vi "Serial Write.vi"(8 "error in (no error)":errorcluster, 10 "Input Command Frame":string, 11 "VISA resource name":refnum<visa-resource-name>) -> (0 "error out":errorcluster, 2 "Bytes Count":i32, 3 "VISA resource name out":refnum<visa-resource-name>)   [LabVIEW 2019, in "BK Precision 178XB Series.lvlib"]
doc: "This VI writes information through the serial port."
uses:
  BK Precision 178XB Series.lvlib
panel:
  in  "Communication Address":u8 max=254 format="%x"
  in  "Start":u8=170 format="%02x"
  in  "Command":u8 format="%02x"
  in  "B01":u8 format="%02x"
  in  "B02":u8 format="%02x"
  in  "B03":u8 format="%02x"
  in  "B04":u8 format="%02x"
  in  "B05":u8 format="%02x"
  in  "B06":u8 format="%02x"
  in  "B07":u8 format="%02x"
  in  "B08":u8 format="%02x"
  in  "B09":u8 format="%02x"
  in  "B10":u8 format="%02x"
  in  "B11":u8 format="%02x"
  in  "B12":u8 format="%02x"
  in  "B13":u8 format="%02x"
  in  "B14":u8 format="%02x"
  in  "B15":u8 format="%02x"
  in  "B16":u8 format="%02x"
  in  "B17":u8 format="%02x"
  in  "B18":u8 format="%02x"
  in  "B19":u8 format="%02x"
  in  "B20":u8 format="%02x"
  in  "B21":u8 format="%02x"
  in  "B22":u8 format="%02x"
  out "CS":u8 format="%02x"
  out "Output Command Frame":u8[](array[numeric])
  # "(c) 2009 B&K PRECISION CORPORATION.  ALL RIGHTS RESERVED."
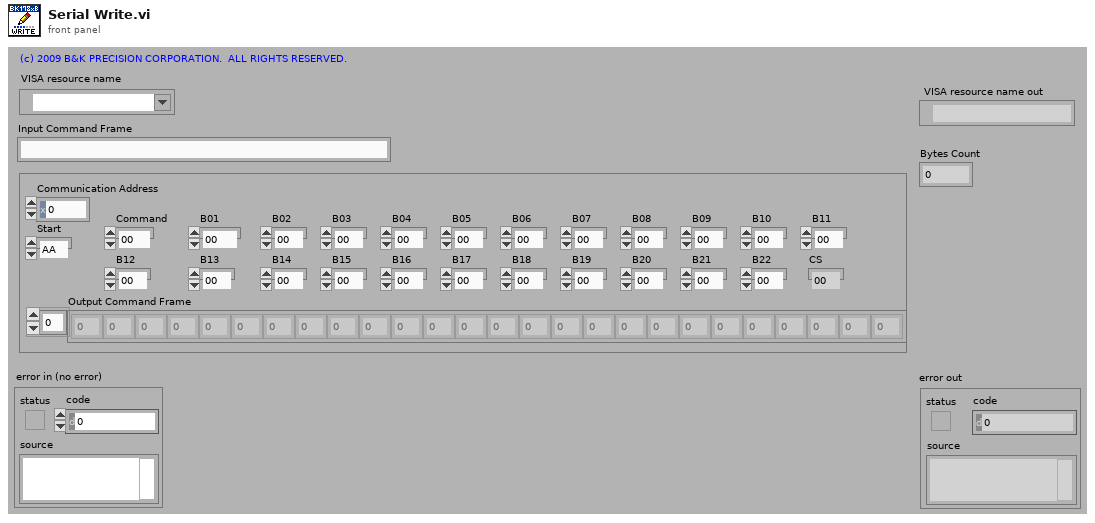
[diagram p1: front panel]
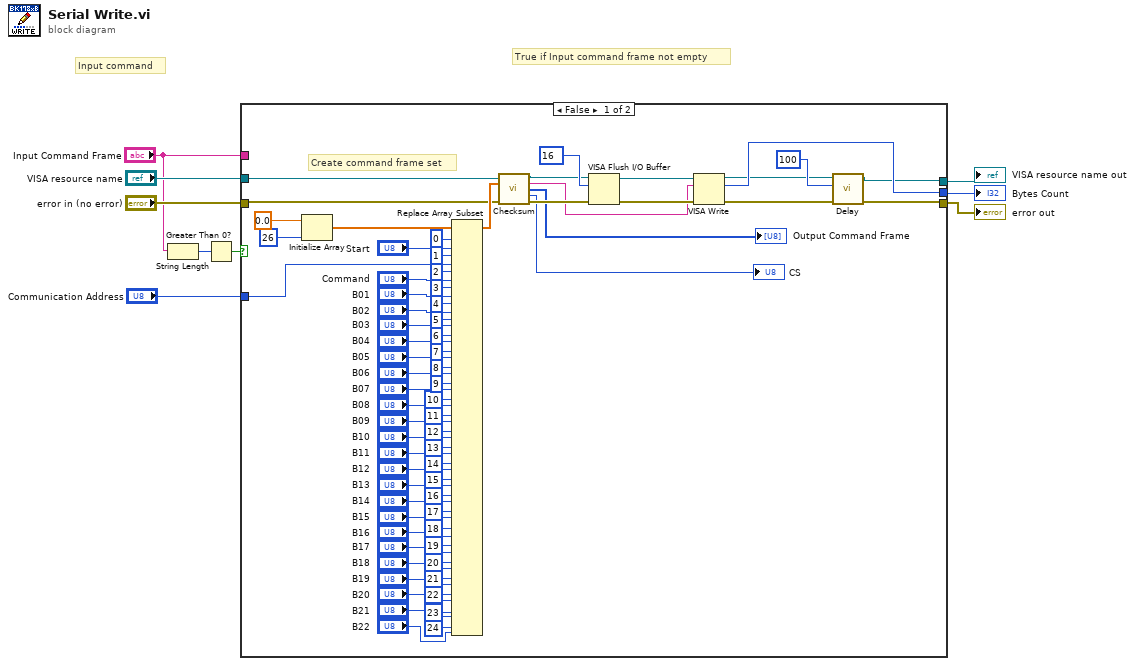
[diagram p0: block diagram]
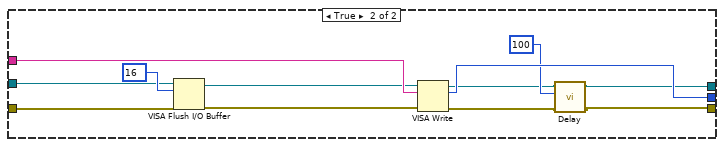
[diagram p2: hidden frame]
diagram:
  # "Input command"
  # "True if Input command frame not empty"
  n1 = String Length(string="Input Command Frame") -> (length=w8:i32)
  n2 = Greater Than 0?(x=w8) -> (x > 0?=w9:bool)
  n3 = case shown="False" w9 {
    tunnel: "VISA resource name" -> [w16 w88]
    tunnel: "error in (no error)" -> [w15 w87]
    tunnel: [w20 w80] -> w5
    tunnel: [w19 w81] -> w1
    tunnel: [w24 w90] -> w4
    tunnel: "Input Command Frame" -> [_ w91]
    tunnel: "Communication Address" -> [w25 _]
    frame False {
      # "Create command frame set"
      n4 = Initialize Array(0.0 ("element"), 26 ("dimension size")) -> (w30:dbl[])
      n5 = Replace Array Subset(array=w30, new element #1="Start", index #1=0 ("index"), new element #2=w25, index #2=1 ("index"), new element #3="Command", index #3=2 ("index"), new element #4="B01", index #4=3 ("index"), new element #5="B02", index #5=4 ("index"), new element #6="B03", index #6=5 ("index"), new element #7="B04", index #7=6 ("index"), new element #8="B05", index #8=7 ("index"), new element #9="B06", index #9=8 ("index"), new element #10="B07", index #10=9 ("index"), new element #11="B08", index #11=10 ("index"), new element #12="B09", index #12=11 ("index"), new element #13="B10", index #13=12 ("index"), new element #14="B11", index #14=13 ("index"), new element #15="B12", index #15=14 ("index"), new element #16="B13", index #16=15 ("index"), new element #17="B14", index #17=16 ("index"), new element #18="B15", index #18=17 ("index"), new element #19="B16", index #19=18 ("index"), new element #20="B17", index #20=19 ("index"), new element #21="B18", index #21=20 ("index"), new element #22="B19", index #22=21 ("index"), new element #23="B20", index #23=22 ("index"), new element #24="B21", index #24=23 ("index"), new element #25="B22", index #25=24 ("index")) -> (w17:dbl[])
      n6 = call "Checksum.vi"("VISA resource name"=w16, "Command Frame Array"=w17, "error in (no error)"=w15) -> ("VISA resource name out"=w14:refnum<visa-resource-name>, "Output String"=w10:string, "Output Array"=→"Output Command Frame":i16[], "Checksum"=→"CS":i16, "error out"=w13:errorcluster)  [unwired: 8 in]
      n7 = VISA Flush I/O Buffer(VISA resource name=w14, mask (16)=u16 16, error in (no error)=w13) -> (VISA resource name out=w28:refnum<visa-resource-name>, error out=w27:errorcluster)
      n8 = VISA Write(VISA resource name=w28, write buffer=w10, error in (no error)=w27) -> (VISA resource name out=w21:refnum<visa-resource-name>, return count=w24:u32, error out=w18:errorcluster)
      n9 = call "Delay.vi"("error in (no error)"=w18, "Delay Value (100)"=100 ("Delay value"), "VISA resource name"=w21) -> ("error out"=w19:errorcluster, "VISA resource name out"=w20:refnum<visa-resource-name>)  [unwired: 7 in]
    }
    frame True {
      n10 = VISA Flush I/O Buffer(VISA resource name=w88, mask (16)=u16 16, error in (no error)=w87) -> (VISA resource name out=w86:refnum<visa-resource-name>, error out=w85:errorcluster)
      n11 = VISA Write(VISA resource name=w86, write buffer=w91, error in (no error)=w85) -> (VISA resource name out=w83:refnum<visa-resource-name>, return count=w90:u32, error out=w82:errorcluster)
      n12 = call "Delay.vi"("error in (no error)"=w82, "Delay Value (100)"=100 ("Delay value"), "VISA resource name"=w83) -> ("error out"=w81:errorcluster, "VISA resource name out"=w80:refnum<visa-resource-name>)  [unwired: 7 in]
    }
  }
  "VISA resource name out" <- w5
  "error out" <- w1
  "Bytes Count" <- w4
